vi "Hough Circles.vi"(4 "Hough Circle Parameters (Default: OpenCV Defaults)":T4={"Param1"=100.0, "Param2"=100.0, "Minimum Radius"=0, "Maximum Radius"=0}, 5 "Minimum Distance":dbl=10.0, 6 "Hough Circle Modes (Default: GRADIENT)":T3, 7 "DP":dbl=1.0, 8 "error in (no error)":errorcluster, 11 "Greyscale Image":refnum<data-value>) -> (0 "error out":errorcluster, 2 "Results":T1[](array[typedef]), 3 "Greyscale Image (Duplicate)":refnum<data-value>)   [LabVIEW 2020, in "g_ar_toolkit.feature_detection.lvlib"]
uses:
  g_ar_toolkit.feature_detection.lvlib
  Hough Circle Parameters.ctl
  Hough Circle Modes.ctl
  Hough Circle Result.ctl
  g_ar_toolkit.common/Image Point (Float).ctl
  Hough Modes.ctl
  g_ar_toolkit.common/g_ar_toolkit.common.lvlib
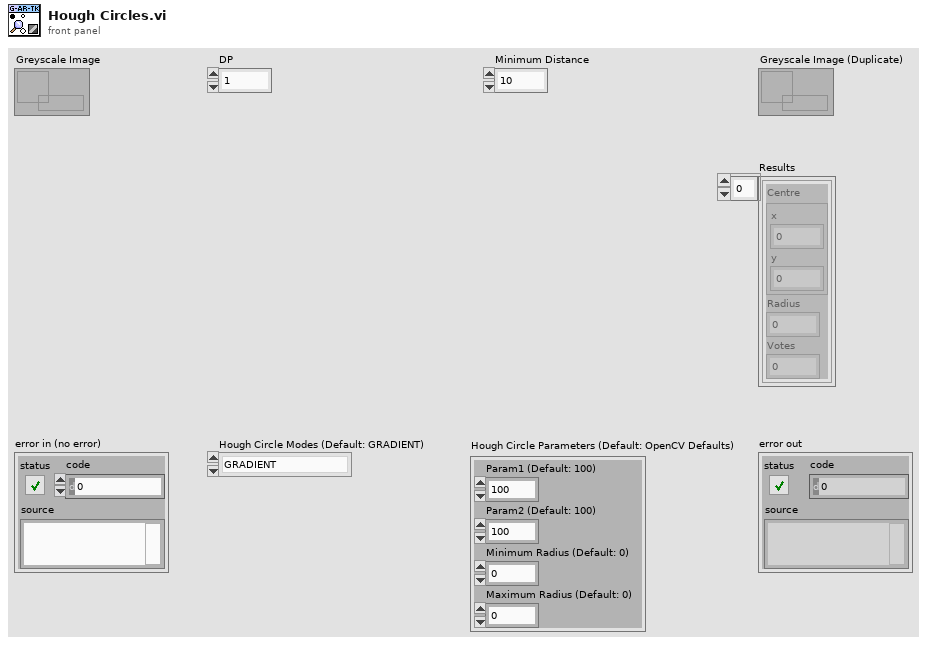
[diagram p1: front panel]
types:
  T1 = typedef "g_ar_toolkit.feature_detection.lvlib/Hough Circle Result.ctl" = cluster{"Centre":T2, "Radius":dbl, "Votes":dbl}
  T2 = typedef "g_ar_toolkit.common.lvlib/Image Point (Float).ctl" = cluster{"x":dbl, "y":dbl}
  T3 = typedef "g_ar_toolkit.feature_detection.lvlib/Hough Circle Modes.ctl" = enum16{"GRADIENT", "GRADIENT_ALT"}
  T4 = typedef "g_ar_toolkit.feature_detection.lvlib/Hough Circle Parameters.ctl" = cluster{"Param1":dbl, "Param2":dbl, "Minimum Radius":i32, "Maximum Radius":i32}
  T5 = typedef "g_ar_toolkit.feature_detection.lvlib/Hough Modes.ctl" = enum16{"STANDARD", "PROBABILISTIC", "MULTI_SCALE", "GRADIENT", "GRADIENT_ALT"}
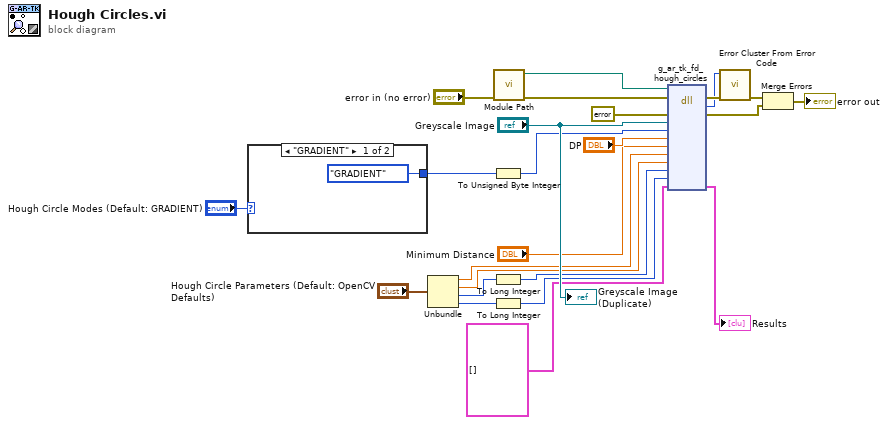
[diagram p0: block diagram]
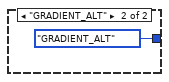
[diagram p2: hidden frame]
diagram:
  n1 = case shown="\"GRADIENT\"" "Hough Circle Modes (Default: GRADIENT)" {
    tunnel: [Hough_Modes."GRADIENT" ("Hough Modes") Hough_Modes."GRADIENT_ALT" ("Hough Modes")] -> w4
    frame "GRADIENT" {
    }
    frame "GRADIENT_ALT" {
    }
  }
  n2 = Unbundle("Hough Circle Parameters (Default: OpenCV Defaults)") -> ("Param1"=w11:dbl, "Param2"=w10:dbl, "Minimum Radius"=w9:i32, "Maximum Radius"=w8:i32)
  n3 = To Unsigned Byte Integer(number=w4) -> (unsigned 8bit integer=w15:u8)
  n4 = To Long Integer(number=w9) -> (32bit integer=w7:i32)
  n5 = To Long Integer(number=w8) -> (32bit integer=w6:i32)
  n6 = call "Module Path.vi"("error in (no error)"="error in (no error)") -> ("error out"=w2:errorcluster, "Path"=w1:path)  [unwired: 9 in]
  n7 = dll-call lib="?" fn="g_ar_tk_fd_hough_circles" ("g_ar_toolkit.*.*:g_ar_tk_image_draw_line")(path in=w1, error in=w2, "error_cluster"=errorcluster {"status"=FALSE, "code"=0, "source"=""} ("error constant"), "EDVR src"="Greyscale Image", "hough_mode"=w15, "dp"="DP", "min_distance"="Minimum Distance", "param1"=w11, "param2"=w10, "min_radius"=w7, "max_radius"=w6, "circles"=T1[] [] ("Array")) -> (error out=w21:errorcluster, "MgErr"=w20:i32, "error_cluster"=w17:errorcluster, "circles"=→"Results":T1[])  [unwired: 9 in, 1 out]
  n8 = call <vilib>:"Error Cluster From Error Code.vi"("error in (no error)"=w21, "error code (0)"=w20) -> ("error out"=w19:errorcluster)  [unwired: 7 in]
  n9 = Merge Errors(w19, w17) -> (→"error out":errorcluster)
  "Greyscale Image (Duplicate)" <- "Greyscale Image"
